vi "质控中断报警全局.vi"() -> ()   [LabVIEW 2016, in "质控单元.lvlib"]
panel:
  out "CODCr中断报警":bool
  out "CODMn中断报警":bool
  out "总氮中断报警":bool
  out "总磷中断报警":bool
  out "氨氮中断报警":bool
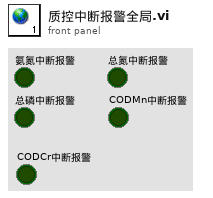
[diagram p1: front panel]
diagram:
